vi "INSERT_CODE.vi"(6 "错误输入":errorcluster, 8 "PRODUCT_ID":string, 9 "CODE_SENSOR":string) -> (0 "错误输出":errorcluster caption="错误输入")   [LabVIEW 2020]
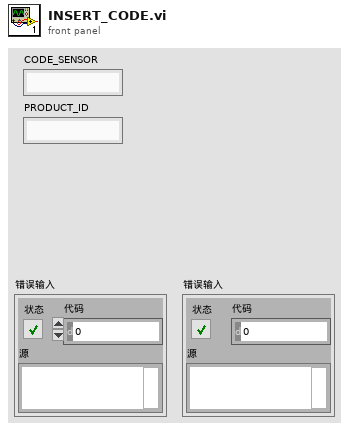
[diagram p1: front panel]
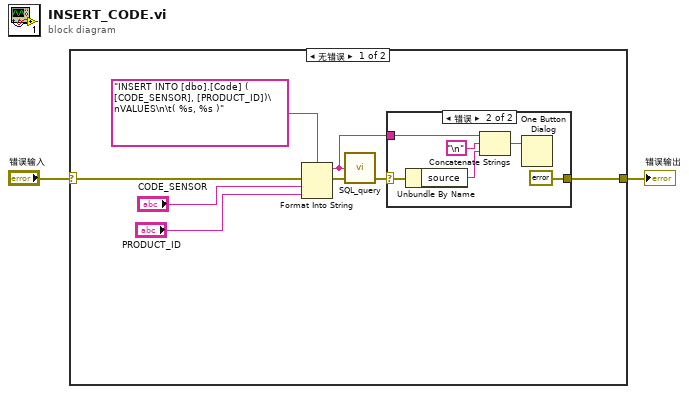
[diagram p0: block diagram]
diagram:
  n1 = case shown="无错误" "错误输入" {
    selector: "错误输入" -> [w9 w18]
    tunnel: [w10 w18] -> w1
    frame No Error {
      n2 = Format Into String(format string="INSERT INTO [dbo].[Code] ( [CODE_SENSOR], [PRODUCT_ID])\nVALUES\n\t( %s, %s )", error in=w9, "CODE_SENSOR", "PRODUCT_ID") -> (resulting string=w4:string, error out=w8:errorcluster)  [unwired: 1 in]
      n3 = call "SQL_query.vi"("error in (no error)"=w8, "SQL query"=w4) -> ("error out"=w5:errorcluster)  [unwired: 1 in, 2 out]
      n4 = case shown="错误" w5 {
        selector: w5 -> [w11 w16]
        tunnel: [w11 errorcluster {"status"=FALSE, "code"=0, "source"=""} ("error IO")] -> w10
        tunnel: w4 -> [_ w15]
        frame No Error {
        }
        frame Error {
          n5 = Unbundle By Name(w16) -> ("source"=w13:string)
          n6 = Concatenate Strings(w15, "\n", w13) -> (w12:string)
          n7 = One Button Dialog(message=w12) -> ()  [unwired: 1 in, 1 out]
        }
      }
    }
    frame Error {
    }
  }
  "错误输出" <- w1
